vi "仪器参数设置.vi"(11 "仪器参数":T1) -> (2 "仪器参数 2":T1, 3 "check？":bool)   [LabVIEW 2016, in "斯坦道总磷.lvlib"]
uses:
  <vilib>/Utility/miscctls.llb/LVPointTypeDef.ctl
  <vilib>/addons/database/Auxilliary.llb/DB Tools DataTypes.ctl
  <vilib>/regexp/Match Regular Expression.xnode
  <vilib>/addons/database/NI_Database_API.lvlib
panel:
  in  "仪器参数表":i32(listbox)
  in  "取消":bool
  in  "确定":bool
  # "仪器参数"
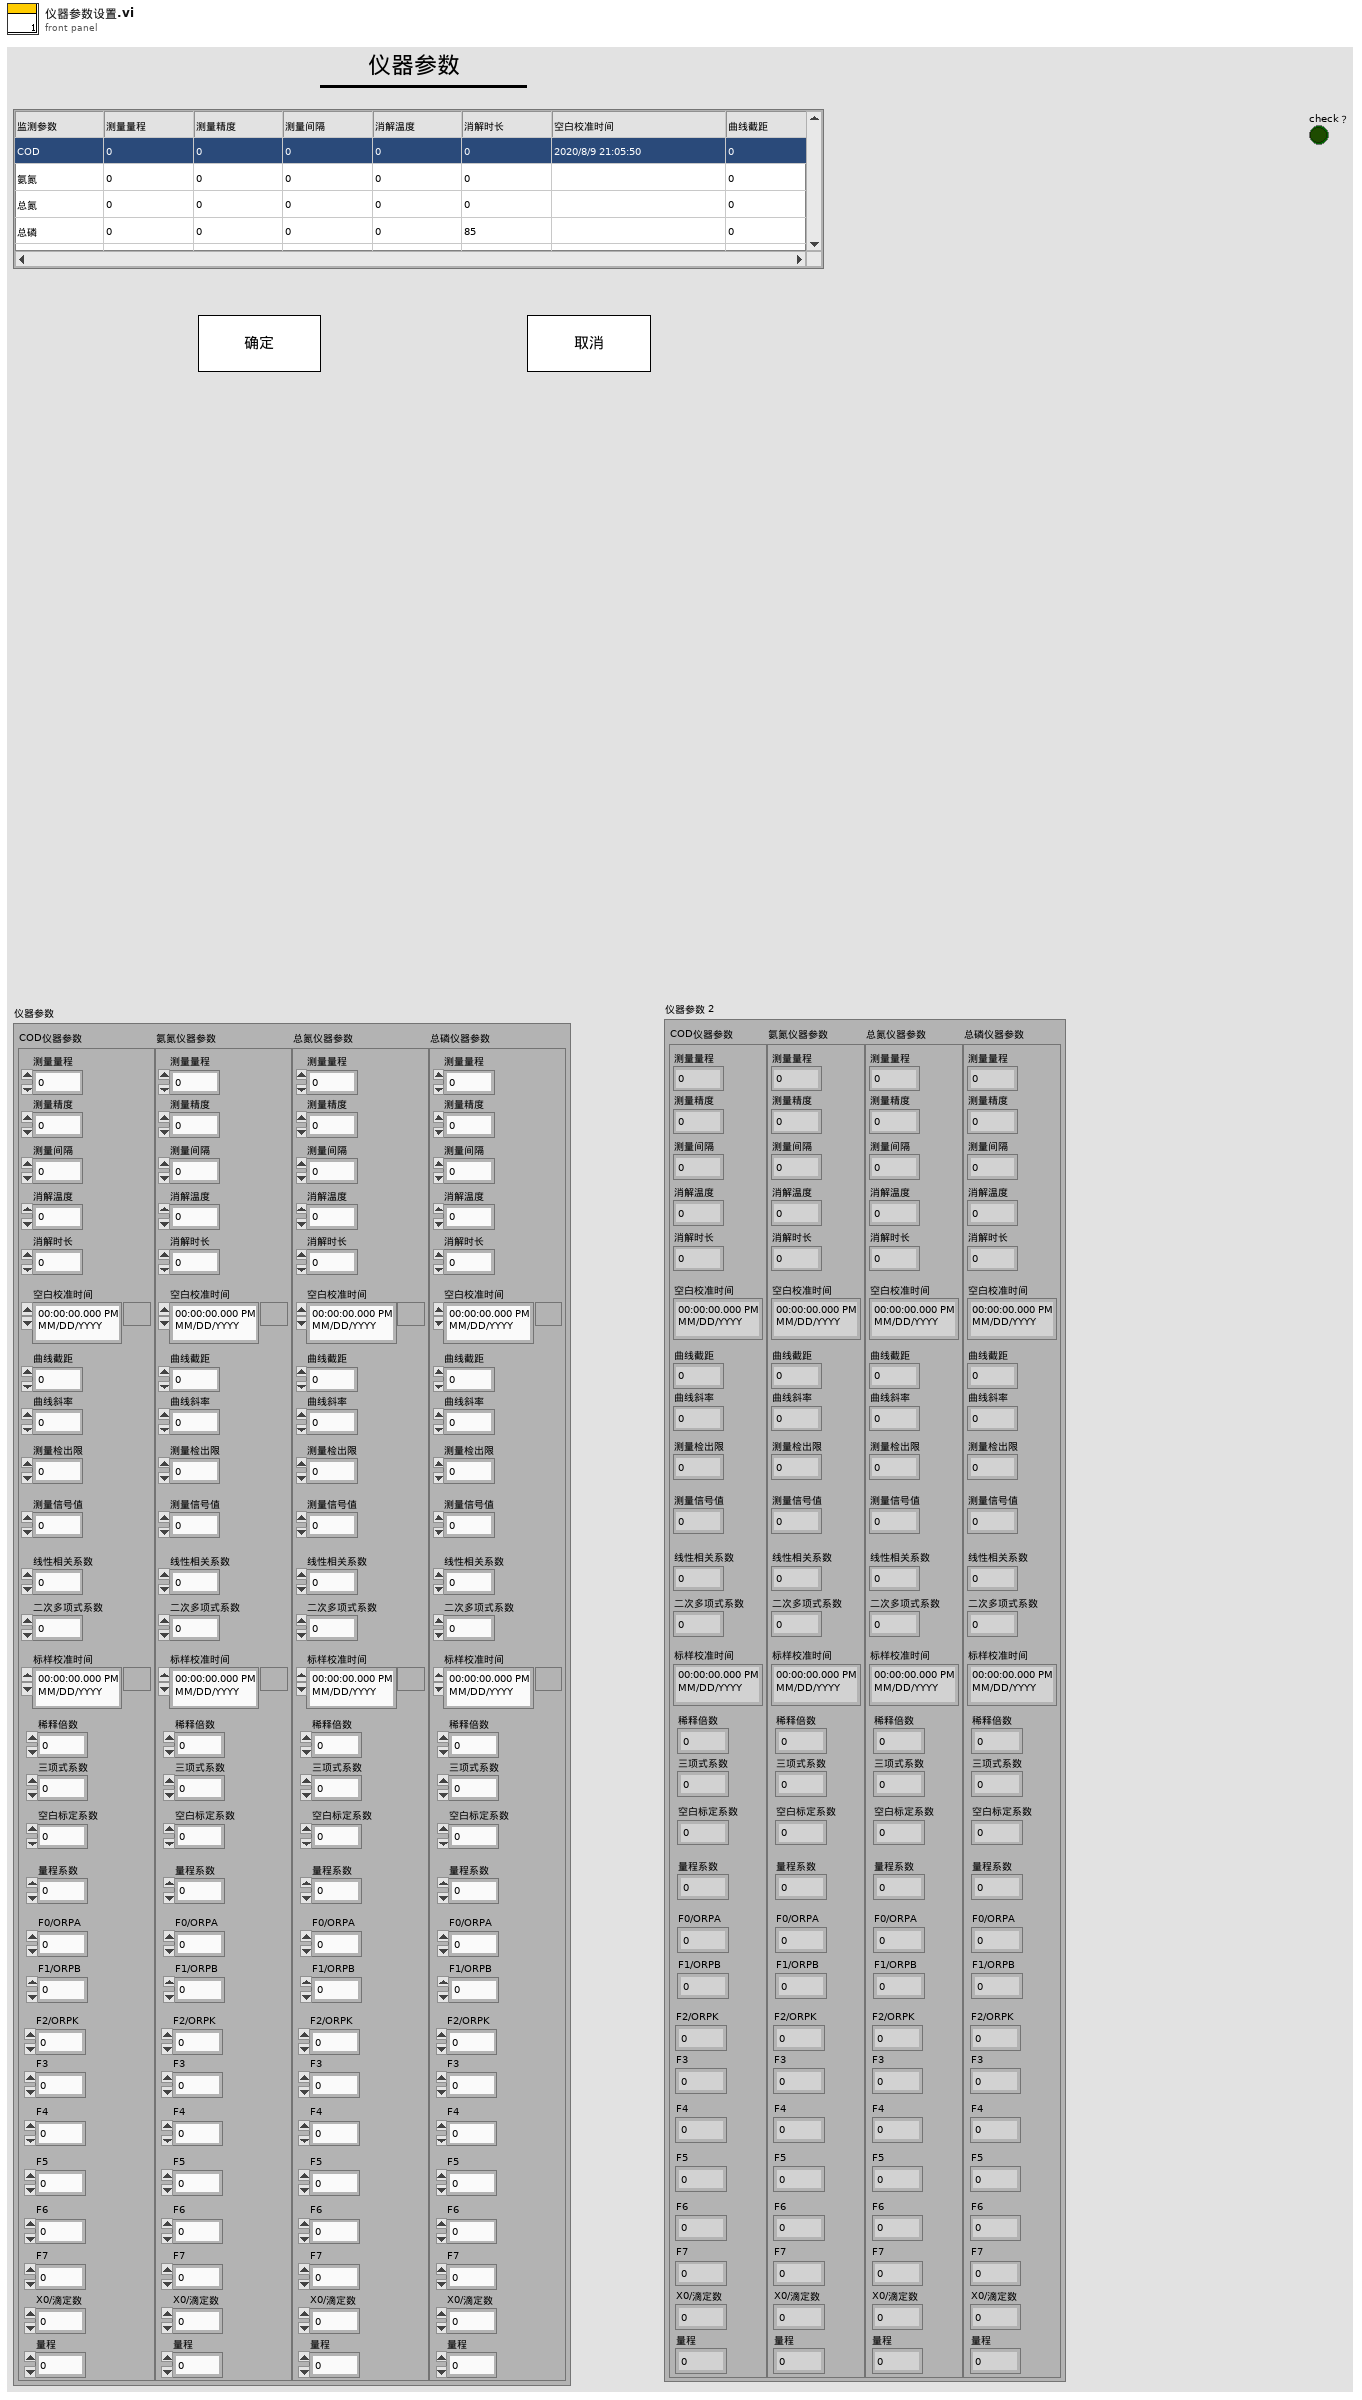
[diagram p1: front panel]
types:
  T1 = cluster{"COD仪器参数":cluster{"测量量程":dbl, "测量精度":dbl, "测量间隔":dbl, "消解温度":dbl, "消解时长":dbl, "空白校准时间":timestamp, "曲线截距":dbl, "曲线斜率":dbl, "测量检出限":dbl, "测量信号值":dbl, "线性相关系数":dbl, "二次多项式系数":dbl, "标样校准时间":timestamp, "稀释倍数":dbl, "三项式系数":dbl, "空白标定系数":dbl, "量程系数":dbl, "F0/ORPA":dbl, "F1/ORPB":dbl, "F2/ORPK":dbl, "F3":dbl, "F4":dbl, "F5":dbl, "F6":dbl, "F7":dbl, "X0/滴定数":dbl, "量程":dbl}, "氨氮仪器参数":cluster{"测量量程":dbl, "测量精度":dbl, "测量间隔":dbl, "消解温度":dbl, "消解时长":dbl, "空白校准时间":timestamp, "曲线截距":dbl, "曲线斜率":dbl, "测量检出限":dbl, "测量信号值":dbl, "线性相关系数":dbl, "二次多项式系数":dbl, "标样校准时间":timestamp, "稀释倍数":dbl, "三项式系数":dbl, "空白标定系数":dbl, "量程系数":dbl, "F0/ORPA":dbl, "F1/ORPB":dbl, "F2/ORPK":dbl, "F3":dbl, "F4":dbl, "F5":dbl, "F6":dbl, "F7":dbl, "X0/滴定数":dbl, "量程":dbl}, "总氮仪器参数":cluster{"测量量程":dbl, "测量精度":dbl, "测量间隔":dbl, "消解温度":dbl, "消解时长":dbl, "空白校准时间":timestamp, "曲线截距":dbl, "曲线斜率":dbl, "测量检出限":dbl, "测量信号值":dbl, "线性相关系数":dbl, "二次多项式系数":dbl, "标样校准时间":timestamp, "稀释倍数":dbl, "三项式系数":dbl, "空白标定系数":dbl, "量程系数":dbl, "F0/ORPA":dbl, "F1/ORPB":dbl, "F2/ORPK":dbl, "F3":dbl, "F4":dbl, "F5":dbl, "F6":dbl, "F7":dbl, "X0/滴定数":dbl, "量程":dbl}, "总磷仪器参数":cluster{"测量量程":dbl, "测量精度":dbl, "测量间隔":dbl, "消解温度":dbl, "消解时长":dbl, "空白校准时间":timestamp, "曲线截距":dbl, "曲线斜率":dbl, "测量检出限":dbl, "测量信号值":dbl, "线性相关系数":dbl, "二次多项式系数":dbl, "标样校准时间":timestamp, "稀释倍数":dbl, "三项式系数":dbl, "空白标定系数":dbl, "量程系数":dbl, "F0/ORPA":dbl, "F1/ORPB":dbl, "F2/ORPK":dbl, "F3":dbl, "F4":dbl, "F5":dbl, "F6":dbl, "F7":dbl, "X0/滴定数":dbl, "量程":dbl}}
  T2 = typedef "NI_Database_API.lvlib/DB Tools DataTypes.ctl" = enum16{"String", "Long (I32)", "Single (SGL)", "Double (DBL)", "Date/Time", "Binary"}
  T3 = typedef "LVPointTypeDef.ctl" = cluster{"Horizontal":i16, "Vertical":i16}
  T4 = typedef "LVPoint32TypeDef.ctl" = cluster{"Horizontal":i32, "Vertical":i32}
  T5 = typedef "LVRowAndColumnTypeDef.ctl" = cluster{"Row":i32, "Column":i32}
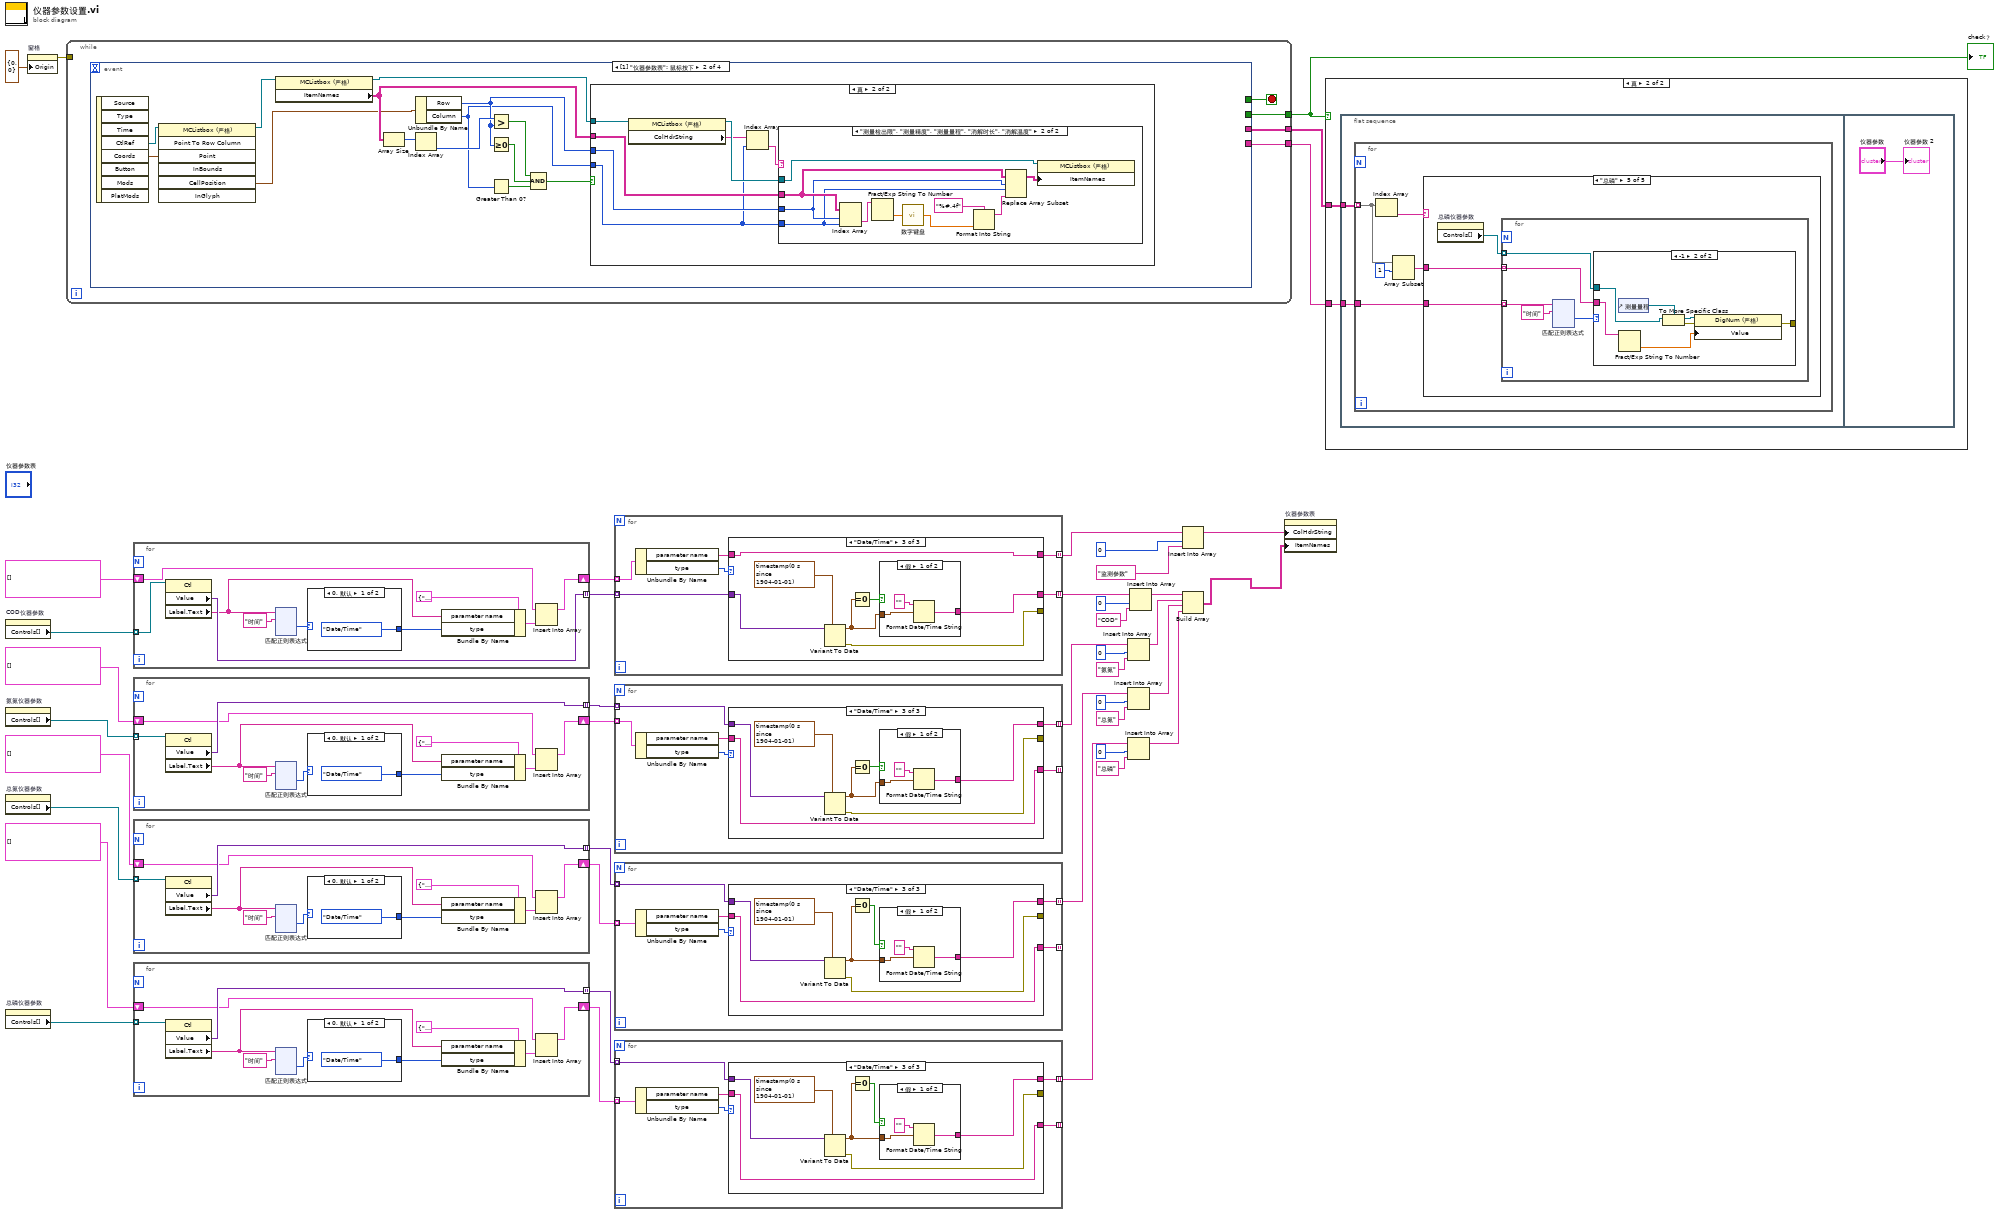
[diagram p0: block diagram]
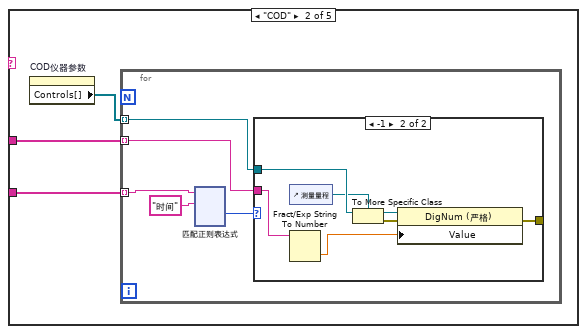
[diagram p4: hidden frame]
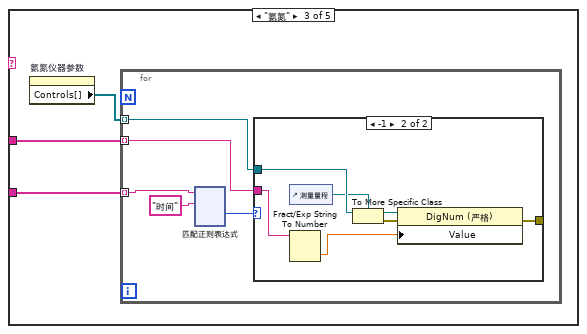
[diagram p6: hidden frame]
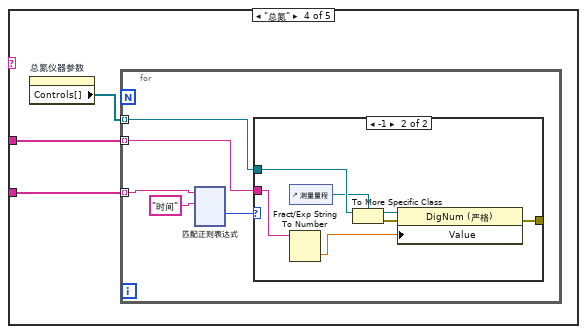
[diagram p8: hidden frame]
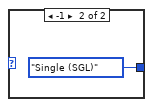
[diagram p11: hidden frame]
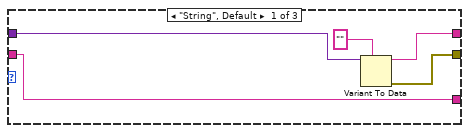
[diagram p12: hidden frame]
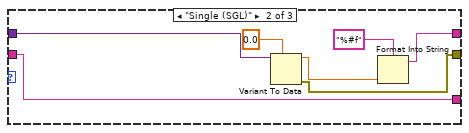
[diagram p13: hidden frame]
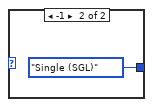
[diagram p15: hidden frame]
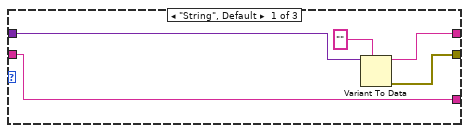
[diagram p16: hidden frame]
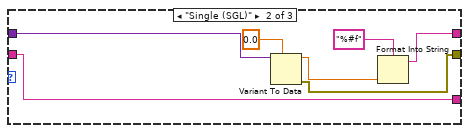
[diagram p17: hidden frame]
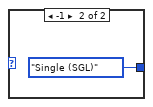
[diagram p19: hidden frame]
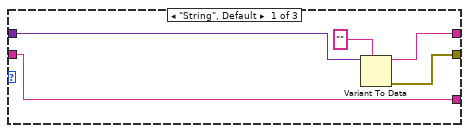
[diagram p20: hidden frame]
diagram:
  n1 = property on="COD仪器参数" class="Clust (严格)"() -> ("Controls[]"=w36:refnum<vi>[])  [unwired: 2 in, 2 out]
  n2 = property on="氨氮仪器参数" class="Clust (严格)"() -> ("Controls[]"=w35:refnum<vi>[])  [unwired: 2 in, 2 out]
  n3 = property on="总氮仪器参数" class="Clust (严格)"() -> ("Controls[]"=w28:refnum<vi>[])  [unwired: 2 in, 2 out]
  n4 = property on="总磷仪器参数" class="Clust (严格)"() -> ("Controls[]"=w27:refnum<vi>[])  [unwired: 2 in, 2 out]
  n5 = property on="窗格" class="Pane"("Origin"=T3 {"Horizontal"=0, "Vertical"=0} ("原点")) -> (error out=w41:errorcluster)  [unwired: 2 in, 1 out]
  n6 = while {
    tunnel: w41 -> [_]
    tunnel: [w45] -> w4
    tunnel: [w44] -> w3
    tunnel: [w43] -> w2
    stop <- w46 stop-if-true
    n7 = event shown="[1] \"仪器参数表\": 鼠标按下" {
      selector: _ -> [_ _ _ _]
      dyn-events: _ -> [_ _ _ _]
      timeout: _ -> [_ _ _ _]
      tunnel: [_ _ TRUE TRUE] -> w46
      tunnel: [_ _ _ "确定"] -> w45
      tunnel: [_ _ _ w80] -> w44
      tunnel: [_ _ _ w79] -> w43
      event Timeout {
        n8 = event-data() -> ()  [unwired: 1 in, 3 out]
      }
      event "仪器参数表": Mouse Down {
        n9 = event-data() -> ("CtlRef"=w60:refnum<vi>, "Coords"=w59:T4)  [unwired: 1 in, 6 out]
        n10 = invoke class="MCListbox (严格)" method="Point To Row Column"(reference=w60, "Point"=w59) -> (reference out=w48:refnum<vi>, "CellPosition"=w47:T5)  [unwired: 5 in, 5 out]
        n11 = property class="MCListbox (严格)"(reference=w48) -> (reference out=w49:refnum<vi>, "ItemNames"=w52:string[][])  [unwired: 1 in, 1 out]
        n12 = Array Size(array=w52) -> (size(s)=w56:i32[])
        n13 = Unbundle By Name(w47) -> ("Row"=w51:i32, "Column"=w50:i32)
        n14 = Index Array(array=w56) -> (element=w55:i32)  [unwired: 1 in]
        n15 = Greater?(x=w55, y=w51) -> (0:w54:bool)
        n16 = Greater Or Equal To 0?(x=w51) -> (x >= 0?=w53:bool)
        n17 = Greater Than 0?(x=w50) -> (x > 0?=w58:bool)
        n18 = Compound Arithmetic op=AND ("复合运算")(w54, w53, w58) -> (w57:bool)
        n19 = case shown="真" w57 {
          tunnel: w52 -> [_ w67]
          tunnel: w51 -> [_ w66]
          tunnel: w50 -> [_ w62]
          tunnel: w49 -> [_ w65]
          frame False {
          }
          frame True {
            n20 = property class="MCListbox (严格)"(reference=w65) -> (reference out=w64:refnum<vi>, "ColHdrString"=w63:string[])  [unwired: 1 in, 1 out]
            n21 = Index Array(array=w63, index=w62) -> (element=w61:string)
            n22 = case shown="\"测量检出限\", \"测量精度\", \"测量量程\", \"消解时长\", \"消解温度\"" w61 {
              tunnel: w67 -> [_ w73]
              tunnel: w66 -> [_ w72]
              tunnel: w62 -> [_ w71]
              tunnel: w64 -> [_ w68]
              frame Default {
              }
              frame "测量检出限", "测量精度", "测量量程", "消解时长", "消解温度" {
                n23 = Index Array(array=w73, index (row)=w72, index (col)=w71) -> (element=w77:string)
                n24 = Fract/Exp String To Number(string=w77) -> (number=w76:dbl)  [unwired: 3 in, 1 out]
                n25 = call "数字键盘.vi"("OldNumber"=w76) -> ("NewNumber"=w75:dbl)
                n26 = Format Into String(format string="%#.4f" ("格式字符串"), w75) -> (resulting string=w70:string)  [unwired: 2 in, 1 out]
                n27 = Replace Array Subset(array=w73, new element=w70, index (row)=w72, index (col)=w71) -> (w69:string[][])
                n28 = property class="MCListbox (严格)"(reference=w68, "ItemNames"=w69) -> ()  [unwired: 1 in, 2 out]
              }
            }
          }
        }
      }
      event "取消": Value Change; Panel Close {
        n29 = event-data() -> ()  [unwired: 1 in, 3 out]
      }
      event "确定": Value Change {
        n30 = event-data() -> ()  [unwired: 1 in, 6 out]
        n31 = property on="仪器参数表" class="MCListbox (严格)"() -> ("ItemNames"=w80:string[][], "ColHdrString"=w79:string[])  [unwired: 2 in, 2 out]
      }
    }
  }
  "check？" <- w4
  n32 = for {
    tunnel: w36 -> [w92] mode=indexing
    tunnel: [w91] -> w40 mode=indexing
    shift-right: [w89] -> w37
    shift-left: cluster{"parameter name":string, "type":T2}[] [] ("parameters out") -> [w90]
    n33 = property class="Ctl"(reference=w92) -> ("Value"=w91:variant, "Label.Text"=w87:string)  [unwired: 1 in, 2 out]
    n34 = xnode "匹配正则表达式"("输入字符串"=w87, "正则表达式"="时间") -> ("匹配后偏移量"=w85:i32)  [unwired: 4 in, 4 out]
    n35 = case shown="0, 默认" w85 {
      tunnel: [DB_Tools_DataTypes."Date/Time" ("type") DB_Tools_DataTypes."Single (SGL)" ("type")] -> w84
      frame 0, Default {
      }
      frame -1 {
      }
    }
    n36 = Bundle By Name(cluster=cluster{"parameter name":string, "type":T2} {"parameter name"="", "type"=enum."String"} ("parameter information"), "parameter name"=w87, "type"=w84) -> (w83:cluster{"parameter name":string, "type":T2})
    n37 = Insert Into Array(array=w90, new element=w83) -> (w89:cluster{"parameter name":string, "type":T2}[])  [unwired: 1 in]
  }
  n38 = for {
    tunnel: w35 -> [w218] mode=indexing
    tunnel: [w217] -> w32 mode=indexing
    shift-right: [w215] -> w34
    shift-left: cluster{"parameter name":string, "type":T2}[] [] ("parameters out") -> [w216]
    n39 = property class="Ctl"(reference=w218) -> ("Value"=w217:variant, "Label.Text"=w213:string)  [unwired: 1 in, 2 out]
    n40 = xnode "匹配正则表达式"("输入字符串"=w213, "正则表达式"="时间") -> ("匹配后偏移量"=w211:i32)  [unwired: 4 in, 4 out]
    n41 = case shown="0, 默认" w211 {
      tunnel: [DB_Tools_DataTypes."Date/Time" ("type") DB_Tools_DataTypes."Single (SGL)" ("type")] -> w210
      frame 0, Default {
      }
      frame -1 {
      }
    }
    n42 = Bundle By Name(cluster=cluster{"parameter name":string, "type":T2} {"parameter name"="", "type"=enum."String"} ("parameter information"), "parameter name"=w213, "type"=w210) -> (w209:cluster{"parameter name":string, "type":T2})
    n43 = Insert Into Array(array=w216, new element=w209) -> (w215:cluster{"parameter name":string, "type":T2}[])  [unwired: 1 in]
  }
  n44 = for {
    tunnel: w28 -> [w344] mode=indexing
    tunnel: [w343] -> w31 mode=indexing
    shift-right: [w341] -> w29
    shift-left: cluster{"parameter name":string, "type":T2}[] [] ("parameters out") -> [w342]
    n45 = property class="Ctl"(reference=w344) -> ("Value"=w343:variant, "Label.Text"=w339:string)  [unwired: 1 in, 2 out]
    n46 = xnode "匹配正则表达式"("输入字符串"=w339, "正则表达式"="时间") -> ("匹配后偏移量"=w337:i32)  [unwired: 4 in, 4 out]
    n47 = case shown="0, 默认" w337 {
      tunnel: [DB_Tools_DataTypes."Date/Time" ("type") DB_Tools_DataTypes."Single (SGL)" ("type")] -> w336
      frame 0, Default {
      }
      frame -1 {
      }
    }
    n48 = Bundle By Name(cluster=cluster{"parameter name":string, "type":T2} {"parameter name"="", "type"=enum."String"} ("parameter information"), "parameter name"=w339, "type"=w336) -> (w335:cluster{"parameter name":string, "type":T2})
    n49 = Insert Into Array(array=w342, new element=w335) -> (w341:cluster{"parameter name":string, "type":T2}[])  [unwired: 1 in]
  }
  n50 = for {
    tunnel: w27 -> [w470] mode=indexing
    tunnel: [w469] -> w24 mode=indexing
    shift-right: [w467] -> w26
    shift-left: cluster{"parameter name":string, "type":T2}[] [] ("parameters out") -> [w468]
    n51 = property class="Ctl"(reference=w470) -> ("Value"=w469:variant, "Label.Text"=w465:string)  [unwired: 1 in, 2 out]
    n52 = xnode "匹配正则表达式"("输入字符串"=w465, "正则表达式"="时间") -> ("匹配后偏移量"=w463:i32)  [unwired: 4 in, 4 out]
    n53 = case shown="0, 默认" w463 {
      tunnel: [DB_Tools_DataTypes."Date/Time" ("type") DB_Tools_DataTypes."Single (SGL)" ("type")] -> w462
      frame 0, Default {
      }
      frame -1 {
      }
    }
    n54 = Bundle By Name(cluster=cluster{"parameter name":string, "type":T2} {"parameter name"="", "type"=enum."String"} ("parameter information"), "parameter name"=w465, "type"=w462) -> (w461:cluster{"parameter name":string, "type":T2})
    n55 = Insert Into Array(array=w468, new element=w461) -> (w467:cluster{"parameter name":string, "type":T2}[])  [unwired: 1 in]
  }
  n56 = for {
    tunnel: w37 -> [w592] mode=indexing
    tunnel: w40 -> [w590] mode=indexing
    tunnel: [w588] -> w38 mode=indexing
    tunnel: [w587] -> w20 mode=indexing
    n57 = Unbundle By Name(w592) -> ("parameter name"=w589:string, "type"=w591:T2)
    n58 = case shown="\"Date/Time\"" w591 {
      tunnel: w590 -> [w596 w604 w611]
      tunnel: w589 -> [w595 w603 w609]
      tunnel: [w595 w603 w609] -> w588
      tunnel: [w594 w598 w607] -> w587
      tunnel: [w593 w602 w608] -> _
      frame "String", Default {
        n59 = Variant To Data(type="", Variant=w596) -> (data=w594:string, error out=w593:errorcluster)  [unwired: 1 in]
      }
      frame "Single (SGL)" {
        n60 = Variant To Data(type=sgl 0.0, Variant=w604) -> (data=w600:sgl, error out=w602:errorcluster)  [unwired: 1 in]
        n61 = Format Into String(format string="%#f" ("格式字符串"), w600) -> (resulting string=w598:string)  [unwired: 2 in, 1 out]
      }
      frame "Date/Time" {
        n62 = Variant To Data(type=timestamp(0 s since 1904-01-01) ("时间标识"), Variant=w611) -> (data=w606:timestamp, error out=w608:errorcluster)  [unwired: 1 in]
        n63 = Equal To 0?(x=w606) -> (x = 0?=w605:bool)
        n64 = case shown="假" w605 {
          tunnel: [w614 _] -> w607
          tunnel: w606 -> [w612 _]
          frame False {
            n65 = Format Date/Time String(time format string (%c)="" ("时间格式字符串(%c)"), seconds (now)=w612) -> (date/time string=w614:string)  [unwired: 1 in]
          }
          frame True {
          }
        }
      }
    }
  }
  n66 = for {
    tunnel: w34 -> [w620] mode=indexing
    tunnel: w32 -> [w618] mode=indexing
    tunnel: [w616] -> _ mode=indexing
    tunnel: [w615] -> w11 mode=indexing
    n67 = Unbundle By Name(w620) -> ("parameter name"=w617:string, "type"=w619:T2)
    n68 = case shown="\"Date/Time\"" w619 {
      tunnel: w618 -> [w624 w632 w639]
      tunnel: w617 -> [w623 w631 w637]
      tunnel: [w623 w631 w637] -> w616
      tunnel: [w622 w626 w635] -> w615
      tunnel: [w621 w630 w636] -> _
      frame "String", Default {
        n69 = Variant To Data(type="", Variant=w624) -> (data=w622:string, error out=w621:errorcluster)  [unwired: 1 in]
      }
      frame "Single (SGL)" {
        n70 = Variant To Data(type=sgl 0.0, Variant=w632) -> (data=w628:sgl, error out=w630:errorcluster)  [unwired: 1 in]
        n71 = Format Into String(format string="%#f" ("格式字符串"), w628) -> (resulting string=w626:string)  [unwired: 2 in, 1 out]
      }
      frame "Date/Time" {
        n72 = Variant To Data(type=timestamp(0 s since 1904-01-01) ("时间标识"), Variant=w639) -> (data=w634:timestamp, error out=w636:errorcluster)  [unwired: 1 in]
        n73 = Equal To 0?(x=w634) -> (x = 0?=w633:bool)
        n74 = case shown="假" w633 {
          tunnel: [w642 _] -> w635
          tunnel: w634 -> [w640 _]
          frame False {
            n75 = Format Date/Time String(time format string (%c)="" ("时间格式字符串(%c)"), seconds (now)=w640) -> (date/time string=w642:string)  [unwired: 1 in]
          }
          frame True {
          }
        }
      }
    }
  }
  n76 = for {
    tunnel: w29 -> [w648] mode=indexing
    tunnel: w31 -> [w646] mode=indexing
    tunnel: [w644] -> _ mode=indexing
    tunnel: [w643] -> w10 mode=indexing
    n77 = Unbundle By Name(w648) -> ("parameter name"=w645:string, "type"=w647:T2)
    n78 = case shown="\"Date/Time\"" w647 {
      tunnel: w646 -> [w652 w660 w667]
      tunnel: w645 -> [w651 w659 w665]
      tunnel: [w651 w659 w665] -> w644
      tunnel: [w650 w654 w663] -> w643
      tunnel: [w649 w658 w664] -> _
      frame "String", Default {
        n79 = Variant To Data(type="", Variant=w652) -> (data=w650:string, error out=w649:errorcluster)  [unwired: 1 in]
      }
      frame "Single (SGL)" {
        n80 = Variant To Data(type=sgl 0.0, Variant=w660) -> (data=w656:sgl, error out=w658:errorcluster)  [unwired: 1 in]
        n81 = Format Into String(format string="%#f" ("格式字符串"), w656) -> (resulting string=w654:string)  [unwired: 2 in, 1 out]
      }
      frame "Date/Time" {
        n82 = Variant To Data(type=timestamp(0 s since 1904-01-01) ("时间标识"), Variant=w667) -> (data=w662:timestamp, error out=w664:errorcluster)  [unwired: 1 in]
        n83 = Equal To 0?(x=w662) -> (x = 0?=w661:bool)
        n84 = case shown="假" w661 {
          tunnel: w662 -> [w670 _]
          tunnel: [w669 _] -> w663
          frame False {
            n85 = Format Date/Time String(time format string (%c)="" ("时间格式字符串(%c)"), seconds (now)=w670) -> (date/time string=w669:string)  [unwired: 1 in]
          }
          frame True {
          }
        }
      }
    }
  }
  n86 = for {
    tunnel: w26 -> [w676] mode=indexing
    tunnel: w24 -> [w674] mode=indexing
    tunnel: [w672] -> _ mode=indexing
    tunnel: [w671] -> w9 mode=indexing
    n87 = Unbundle By Name(w676) -> ("parameter name"=w673:string, "type"=w675:T2)
    n88 = case shown="\"Date/Time\"" w675 {
      tunnel: w674 -> [w680 w688 w695]
      tunnel: w673 -> [w679 w687 w693]
      tunnel: [w679 w687 w693] -> w672
      tunnel: [w678 w682 w691] -> w671
      tunnel: [w677 w686 w692] -> _
      frame "String", Default {
        n89 = Variant To Data(type="", Variant=w680) -> (data=w678:string, error out=w677:errorcluster)  [unwired: 1 in]
      }
      frame "Single (SGL)" {
        n90 = Variant To Data(type=sgl 0.0, Variant=w688) -> (data=w684:sgl, error out=w686:errorcluster)  [unwired: 1 in]
        n91 = Format Into String(format string="%#f" ("格式字符串"), w684) -> (resulting string=w682:string)  [unwired: 2 in, 1 out]
      }
      frame "Date/Time" {
        n92 = Variant To Data(type=timestamp(0 s since 1904-01-01) ("时间标识"), Variant=w695) -> (data=w690:timestamp, error out=w692:errorcluster)  [unwired: 1 in]
        n93 = Equal To 0?(x=w690) -> (x = 0?=w689:bool)
        n94 = case shown="假" w689 {
          tunnel: w690 -> [w698 _]
          tunnel: [w697 _] -> w691
          frame False {
            n95 = Format Date/Time String(time format string (%c)="" ("时间格式字符串(%c)"), seconds (now)=w698) -> (date/time string=w697:string)  [unwired: 1 in]
          }
          frame True {
          }
        }
      }
    }
  }
  n96 = Insert Into Array(array=w11, index=0 ("索引"), new element="氨氮" ("新元素/子数组")) -> (w7:string[])
  n97 = Insert Into Array(array=w10, index=0 ("索引"), new element="总氮" ("新元素/子数组")) -> (w6:string[])
  n98 = Insert Into Array(array=w9, index=0 ("索引"), new element="总磷" ("新元素/子数组")) -> (w5:string[])
  n99 = Insert Into Array(array=w20, index=0 ("索引"), new element="COD" ("新元素/子数组")) -> (w8:string[])
  n100 = Insert Into Array(array=w38, index=0 ("索引"), new element="监测参数" ("新元素/子数组")) -> (w23:string[])
  n101 = Build Array(w8, w7, w6, w5) -> (w1:string[][])
  n102 = property on="仪器参数表" class="MCListbox (严格)"("ColHdrString"=w23, "ItemNames"=w1) -> ()  [unwired: 2 in, 2 out]
  n103 = case shown="真" w4 {
    tunnel: w3 -> [_ w700]
    tunnel: w2 -> [_ w699]
    frame False {
    }
    frame True {
      n104 = flat-sequence {
        tunnel: w700 -> [w702]
        tunnel: w699 -> [w701]
        frame #0 {
          n105 = for {
            tunnel: w702 -> [w706] mode=indexing
            tunnel: w701 -> [w703]
            n106 = Index Array(array=w706) -> (element=w707:string)  [unwired: 1 in]
            n107 = Array Subset(array=w706, index=1 ("索引")) -> (w704:string[])  [unwired: 1 in]
            n108 = case shown="\"总磷\"" w707 {
              tunnel: w704 -> [_ w710 w839 w968 w1097]
              tunnel: w703 -> [_ w709 w838 w967 w1096]
              frame Default {
              }
              frame "COD" {
                n109 = property on="COD仪器参数" class="Clust (严格)"() -> ("Controls[]"=w708:refnum<vi>[])  [unwired: 2 in, 2 out]
                n110 = for {
                  tunnel: w710 -> [w711] mode=indexing
                  tunnel: w709 -> [w715] mode=indexing
                  tunnel: w708 -> [w712] mode=indexing
                  n111 = xnode "匹配正则表达式"("输入字符串"=w715, "正则表达式"="时间") -> ("匹配后偏移量"=w713:i32)  [unwired: 4 in, 4 out]
                  n112 = case shown="-1" w713 {
                    tunnel: w712 -> [_ w722]
                    tunnel: w711 -> [_ w719]
                    tunnel: [_ w716] -> _
                    frame 0, Default {
                    }
                    frame -1 {
                      n113 = control-ref of="测量量程"() -> (w720:refnum<vi>)
                      n114 = Fract/Exp String To Number(string=w719) -> (number=w718:dbl)  [unwired: 3 in, 1 out]
                      n115 = To More Specific Class(target class=w720, reference=w722) -> (specific class reference=w721:refnum<vi>, error out=w717:errorcluster)  [unwired: 1 in]
                      n116 = property class="DigNum (严格)"(reference=w721, error in=w717, "Value"=w718) -> (error out=w716:errorcluster)  [unwired: 1 out]
                    }
                  }
                }
              }
              frame "氨氮" {
                n117 = property on="氨氮仪器参数" class="Clust (严格)"() -> ("Controls[]"=w837:refnum<vi>[])  [unwired: 2 in, 2 out]
                n118 = for {
                  tunnel: w839 -> [w840] mode=indexing
                  tunnel: w838 -> [w844] mode=indexing
                  tunnel: w837 -> [w841] mode=indexing
                  n119 = xnode "匹配正则表达式"("输入字符串"=w844, "正则表达式"="时间") -> ("匹配后偏移量"=w842:i32)  [unwired: 4 in, 4 out]
                  n120 = case shown="-1" w842 {
                    tunnel: w841 -> [_ w851]
                    tunnel: w840 -> [_ w848]
                    tunnel: [_ w845] -> _
                    frame 0, Default {
                    }
                    frame -1 {
                      n121 = control-ref of="测量量程"() -> (w849:refnum<vi>)
                      n122 = Fract/Exp String To Number(string=w848) -> (number=w847:dbl)  [unwired: 3 in, 1 out]
                      n123 = To More Specific Class(target class=w849, reference=w851) -> (specific class reference=w850:refnum<vi>, error out=w846:errorcluster)  [unwired: 1 in]
                      n124 = property class="DigNum (严格)"(reference=w850, error in=w846, "Value"=w847) -> (error out=w845:errorcluster)  [unwired: 1 out]
                    }
                  }
                }
              }
              frame "总氮" {
                n125 = property on="总氮仪器参数" class="Clust (严格)"() -> ("Controls[]"=w966:refnum<vi>[])  [unwired: 2 in, 2 out]
                n126 = for {
                  tunnel: w968 -> [w969] mode=indexing
                  tunnel: w967 -> [w973] mode=indexing
                  tunnel: w966 -> [w970] mode=indexing
                  n127 = xnode "匹配正则表达式"("输入字符串"=w973, "正则表达式"="时间") -> ("匹配后偏移量"=w971:i32)  [unwired: 4 in, 4 out]
                  n128 = case shown="-1" w971 {
                    tunnel: w970 -> [_ w980]
                    tunnel: w969 -> [_ w977]
                    tunnel: [_ w974] -> _
                    frame 0, Default {
                    }
                    frame -1 {
                      n129 = control-ref of="测量量程"() -> (w978:refnum<vi>)
                      n130 = Fract/Exp String To Number(string=w977) -> (number=w976:dbl)  [unwired: 3 in, 1 out]
                      n131 = To More Specific Class(target class=w978, reference=w980) -> (specific class reference=w979:refnum<vi>, error out=w975:errorcluster)  [unwired: 1 in]
                      n132 = property class="DigNum (严格)"(reference=w979, error in=w975, "Value"=w976) -> (error out=w974:errorcluster)  [unwired: 1 out]
                    }
                  }
                }
              }
              frame "总磷" {
                n133 = property on="总磷仪器参数" class="Clust (严格)"() -> ("Controls[]"=w1095:refnum<vi>[])  [unwired: 2 in, 2 out]
                n134 = for {
                  tunnel: w1097 -> [w1098] mode=indexing
                  tunnel: w1096 -> [w1102] mode=indexing
                  tunnel: w1095 -> [w1099] mode=indexing
                  n135 = xnode "匹配正则表达式"("输入字符串"=w1102, "正则表达式"="时间") -> ("匹配后偏移量"=w1100:i32)  [unwired: 4 in, 4 out]
                  n136 = case shown="-1" w1100 {
                    tunnel: w1099 -> [_ w1109]
                    tunnel: w1098 -> [_ w1106]
                    tunnel: [_ w1103] -> _
                    frame 0, Default {
                    }
                    frame -1 {
                      n137 = control-ref of="测量量程"() -> (w1107:refnum<vi>)
                      n138 = Fract/Exp String To Number(string=w1106) -> (number=w1105:dbl)  [unwired: 3 in, 1 out]
                      n139 = To More Specific Class(target class=w1107, reference=w1109) -> (specific class reference=w1108:refnum<vi>, error out=w1104:errorcluster)  [unwired: 1 in]
                      n140 = property class="DigNum (严格)"(reference=w1108, error in=w1104, "Value"=w1105) -> (error out=w1103:errorcluster)  [unwired: 1 out]
                    }
                  }
                }
              }
            }
          }
        }
        frame #1 {
          "仪器参数 2" <- "仪器参数"
        }
      }
    }
  }
